vi "Event handler-Number of planes change.vi"(8 "error in (no error)":errorcluster) -> (0 "error out":errorcluster)   [LabVIEW 2020]
uses:
  Typedefs/Read Write Enum.ctl
  Global Variables/gl_UI Ctrl Refs.vi
  Global Variables/General Globals.vi
panel:
  out "Z-stop out (um)":dbl
  out "Z-start out (um)":dbl
  out "Adjusted absolute difference (um)":dbl
  out "Exact multiple?":bool
  out "Verified diffrence (um)":dbl
  out "Initial absolute difference (um)":dbl
  out "Z-stop (um)":dbl
  out "Z-start (um)":dbl
  out "Resulting Z Planes(um)":dbl[](array[numeric])
  out "Resulting number of planes":i32
  out "Z-step (um)":dbl
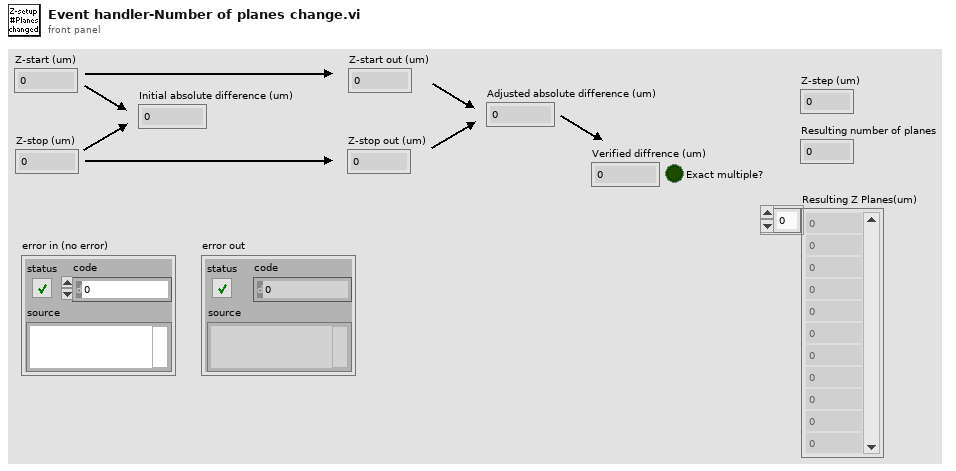
[diagram p1: front panel]
types:
  T1 = typedef "Read Write Enum.ctl" = enum16{"Read", "Write"}
  T2 = typedef "UI ctrl refs cluster.ctl" = cluster{"Top level VI path":path, "Top level VI ref":refnum<vi>, "User menu ref":refnum<k9>, "Sub Panel control":refnum<vi>, "Imaging Param Tab":refnum<vi>, "Occurrence-Start drivers":refnum<k4>, "Occurrence-Speed logging initialised":refnum<k4>, "Occurrence-XYZ stage initialised":refnum<k4>, "Exit button":refnum<vi>, "Status ind":refnum<vi>, "Set as origin":refnum<vi>, "Speed Logging":refnum<vi>, "Time Lapse":refnum<vi>, "Live Imaging":refnum<vi>, "AOL Z Stack":refnum<vi>, "Motor Z Stack":refnum<vi>, "Funct Acq button":refnum<vi>, "Hard Shutter":refnum<vi>, "Virtual Shutter":refnum<vi>, "Laser Power":refnum<vi>, "AOL Mode":refnum<vi>, "Frame Size":refnum<vi>, "Field of View":refnum<vi>, "Dwell Time":refnum<vi>, "Zoom":refnum<vi>, "AOL Z":refnum<vi>, "Objective":refnum<vi>, "Axis":refnum<vi>, "Paths & Names":refnum<vi>, "Experiment folder path (ind.)":refnum<vi>, "Last State (Ind.)":refnum<vi>, "Averages":refnum<vi>, "Angle (degrees)":refnum<vi>, "X centre":refnum<vi>, "Y centre":refnum<vi>, "Plane Mode":refnum<vi>, "# Planes":refnum<vi>, "Z Start":refnum<vi>, "Z Stop":refnum<vi>, "Z Step":refnum<vi>, "PMT 1":refnum<vi>, "PMT 2":refnum<vi>, "Stage XYZ Position":refnum<vi>, "Pockels@Z Start":refnum<vi>, "Pockels@Z Stop":refnum<vi>, "Obtain Z Start":refnum<vi>, "Obtain Z Stop":refnum<vi>, "Live stim.trig.period":refnum<vi>, "Live stim.trig.enable":refnum<vi>, "Movement Correction":refnum<vi>, "Load Reference Image":refnum<vi>, "XY Stage Move":refnum<vi>, "MovCor Cluster":refnum<vi>, "RefDAQParam":refnum<vi>, "Funct. Acq. Pockels Modulation":refnum<vi>, "Ref Laser Power":refnum<vi>, "Enable Video Recording":refnum<vi>, "Video Record-Live Imaging":refnum<vi>, "Video Record-Funct acq":refnum<vi>, "Reference Source":refnum<vi>, "AOL Z-stack Chirps Ready (ind)":refnum<vi>, "Target time between mov.cor. ref triggers (ms)":refnum<vi>, "Funct. Acq. Ref frame save":refnum<vi>, "Tracking button":refnum<vi>, "Show ref plots window":refnum<vi>, "Center freq ind (nm)":refnum<vi>, "Pickup mode (ind)":refnum<vi>, "Logging queue (ind)":refnum<vi>, "Back aperture power (ind.)":refnum<vi>, "Power after objective (ind.)":refnum<vi>, "Switch user":refnum<vi>, "Ls1 Conn. Status":refnum<vi>, "Ls1Tuning Status":refnum<vi>, "Ls1 Faults":refnum<vi>, "Ls1 Connection":refnum<vi>, "Ls1 Mode":refnum<vi>, "Ls1 POWER [mW]":refnum<vi>, "Ls1Shutter":refnum<vi>, "Ls1 Wavelength":refnum<vi>, "Ls1 Note":refnum<vi>, "Ls1 Confirm Wav":refnum<vi>, "Ls1 PreChrp Prism1":refnum<vi>, "Ls1 PreChrp Prism2":refnum<vi>, "Ls1 wav top Ind":refnum<vi>, "Ls1 power top Ind":refnum<vi>, "Ls1 Pump peak Hold":refnum<vi>, "Ls1 Status Ind":refnum<vi>, "Ls1 wav cancel":refnum<vi>, "Experiment Type":refnum<vi>, "Biology Information":refnum<vi>, "Camera recording status":refnum<vi>}
  T3 = cluster{"ZStack":cluster{"Zstart":dbl, "Zstop":dbl, "Zstep":dbl}, "Laser Power %":cluster{"@ Start":dbl, "@ Stop":dbl}}
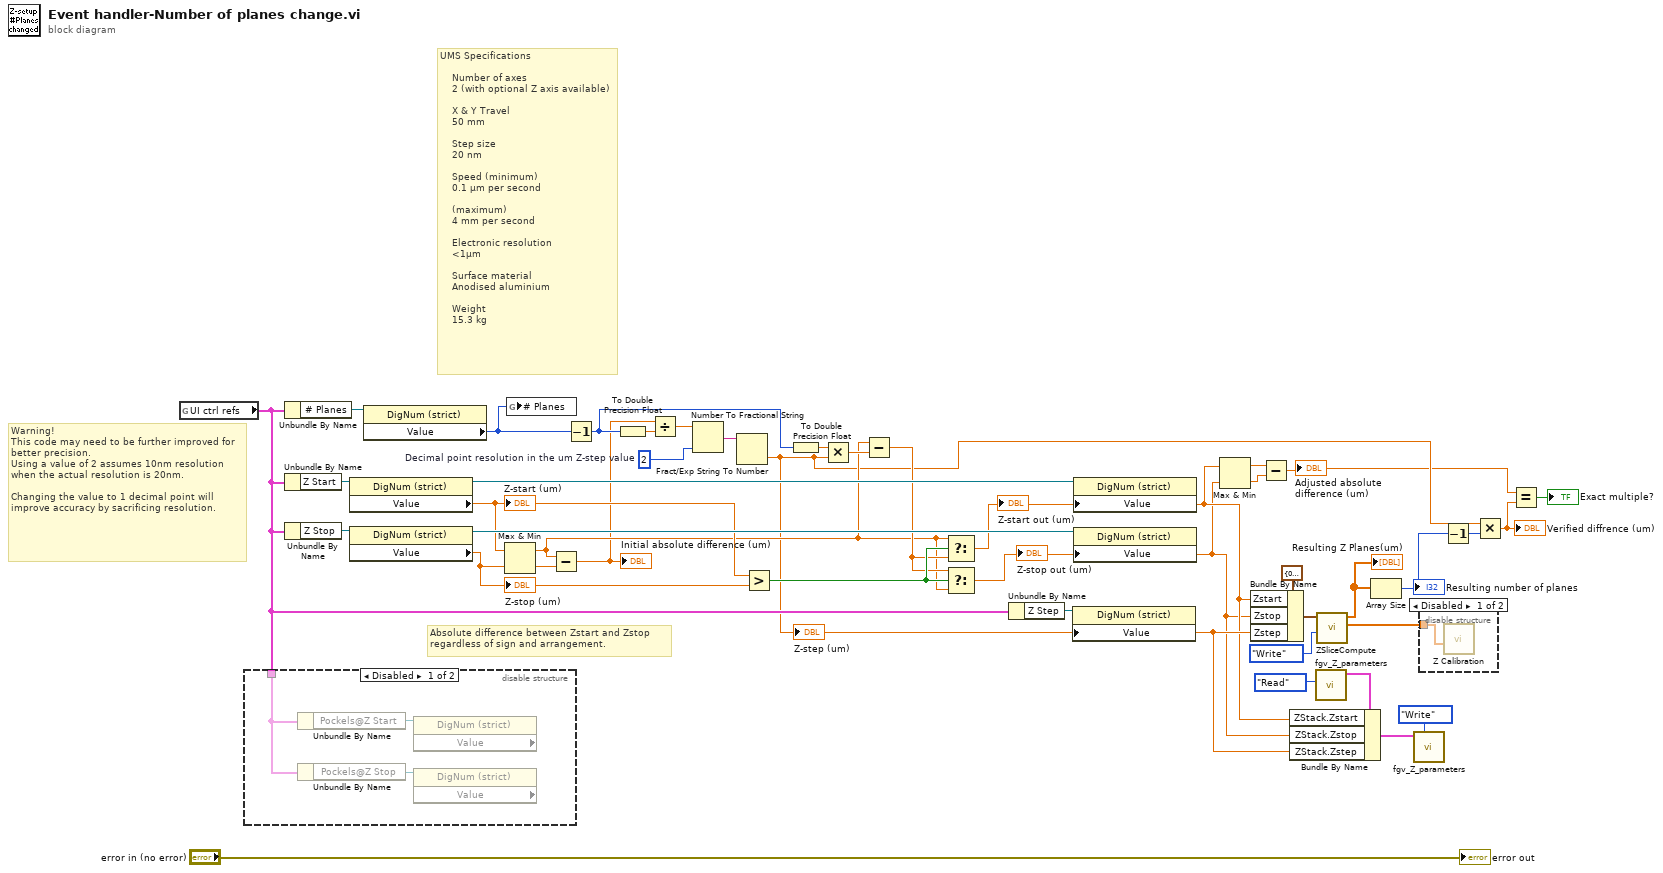
[diagram p0: block diagram]
diagram:
  w27 = i16 2  # Decimal point resolution in the um Z-step value
  # "Warning!\nThis code may need to be further improved for better precision.\nUsing a value of 2 assumes 10nm resolution when the actual resolution is 20nm.\n\nChanging the value to 1 decimal point will improve accuracy by sacrificing resolution."
  # "UMS Specifications\n\n    Number of axes\n    2 (with optional Z axis available)\n\n    X & Y Travel\n    50 mm\n\n    Step size\n    20 nm\n\n    Speed (minimum)\n    0.1 µm per second\n\n    (maximum)\n    4 mm per second\n\n    Electronic resolution\n    <1µm\n\n    Surface material\n    Anodised aluminium\n\n    Weight\n    15.3 kg"
  # "Absolute difference between Zstart and Zstop\nregardless of sign and arrangement."
  n1 = global read "gl_UI Ctrl Refs.vi" "UI ctrl refs"() -> (w42:T2)
  n2 = disable-structure shown="Disabled" {
    disable-tunnel: w42 -> [w45 _]
    frame Disabled {
      n3 = Unbundle By Name(w45) -> ("Pockels@Z Start"=w44:refnum<vi>)
      n4 = Unbundle By Name(w45) -> ("Pockels@Z Stop"=w43:refnum<vi>)
      n5 = property on="Property Node" class="DigNum (strict)" props=["Value"](reference=w44) -> ()  [unwired: 1 in, 3 out]
      n6 = property on="Property Node" class="DigNum (strict)" props=["Value"](reference=w43) -> ()  [unwired: 1 in, 3 out]
    }
    frame Enabled {
    }
  }
  n7 = Unbundle By Name(w42) -> ("# Planes"=w30:refnum<vi>)
  n8 = Unbundle By Name(w42) -> ("Z Start"=w33:refnum<vi>)
  n9 = Unbundle By Name(w42) -> ("Z Stop"=w32:refnum<vi>)
  n10 = property on="Property Node" class="DigNum (strict)"(reference=w33) -> (reference out=w17:refnum<vi>, "Value"=w18:dbl)  [unwired: 1 in, 1 out]
  "Z-start (um)" <- w18
  n11 = property on="Property Node" class="DigNum (strict)"(reference=w32) -> (reference out=w23:refnum<vi>, "Value"=w21:dbl)  [unwired: 1 in, 1 out]
  "Z-stop (um)" <- w21
  n12 = property on="Property Node" class="DigNum (strict)"(reference=w30) -> ("Value"=w2:u16)  [unwired: 1 in, 2 out]
  n13 = Max & Min(x=w18, y=w21) -> (max(x,y)=w14:dbl, min(x,y)=w19:dbl)
  n14 = global write "General Globals.vi" "# Planes"(w2) -> ()
  n15 = Subtract(x=w14, y=w19) -> (x-y=w8:dbl)
  "Initial absolute difference (um)" <- w8
  n16 = Decrement(x=w2) -> (x-1=w22:u16)
  n17 = To Double Precision Float(number=w22) -> (double precision float=w28:dbl)
  n18 = Divide(x=w8, y=w28) -> (x/y=w26:dbl)
  n19 = Number To Fractional String(number=w26, precision (6)=w27) -> (F-format string=w25:string)  [unwired: 2 in]
  n20 = Fract/Exp String To Number(string=w25) -> (number=w12:dbl)  [unwired: 3 in, 1 out]
  "Z-step (um)" <- w12
  n21 = Greater?(x=w18, y=w21) -> (0:w16:bool)
  n22 = To Double Precision Float(number=w22) -> (double precision float=w24:dbl)
  n23 = Multiply(x=w24, y=w12) -> (x*y=w20:dbl)
  n24 = Subtract(x=w14, y=w20) -> (x-y=w15:dbl)
  n25 = Select(t=w14, s=w16, f=w15) -> (s? t:f=w4:dbl)
  "Z-start out (um)" <- w4
  n26 = Select(t=w15, s=w16, f=w14) -> (s? t:f=w3:dbl)
  "Z-stop out (um)" <- w3
  n27 = Unbundle By Name(w42) -> ("Z Step"=w31:refnum<vi>)
  n28 = property on="Property Node" class="DigNum (strict)"(reference=w31, "Value"=w12) -> ()  [unwired: 1 in, 2 out]
  n29 = property on="Property Node" class="DigNum (strict)"(reference=w17, "Value"=w4) -> ()  [unwired: 1 in, 2 out]
  n30 = property on="Property Node" class="DigNum (strict)"(reference=w23, "Value"=w3) -> ()  [unwired: 1 in, 2 out]
  n31 = Max & Min(x=w4, y=w3) -> (max(x,y)=w7:dbl, min(x,y)=w6:dbl)
  n32 = Bundle By Name(cluster=cluster{"Zstart":dbl, "Zstop":dbl, "Zstep":dbl} {"Zstart"=0.0, "Zstop"=0.0, "Zstep"=0.0} ("ZStack"), "Zstart"=w4, "Zstop"=w3, "Zstep"=w12) -> (w40:cluster{"Zstart":dbl, "Zstop":dbl, "Zstep":dbl})
  n33 = Subtract(x=w7, y=w6) -> (x-y=w5:dbl)
  "Adjusted absolute difference (um)" <- w5
  n34 = call "fgv_Z_parameters.vi"("Function"=enum16{"Intialize", "Write", "Read", "Clear"}."Read") -> ("Z Parameters"=w35:T3)  [unwired: 9 in, 1 out]
  n35 = Bundle By Name(cluster=w35, "ZStack.Zstart"=w4, "ZStack.Zstop"=w3, "ZStack.Zstep"=w12) -> (w34:T3)
  n36 = call "ZSliceCompute.vi"("Function"=Read_Write_Enum."Write", "ZStack (um)"=w40) -> ("AOL Z Planes(um)"=w38:dbl[], "Motor Z Planes(um)"=w39:dbl[])  [unwired: 6 in, 2 out]
  "Resulting Z Planes(um)" <- w39
  n37 = Array Size(array=w39) -> (size(s)=w13:i32)
  "Resulting number of planes" <- w13
  n38 = call "fgv_Z_parameters.vi"("Function"=enum16{"Intialize", "Write", "Read", "Clear"}."Write", "Z Parameters"=w34) -> ()  [unwired: 8 in, 2 out]
  n39 = disable-structure "Diagram Disable Structure" shown="Disabled" {
    disable-tunnel: w38 -> [w46 _]
    frame Disabled {
      n40 = call "Z Calibration.vi"("Z Planes"=w46) -> ()  [unwired: 7 in, 4 out]
    }
    frame Enabled {
    }
  }
  n41 = Decrement(x=w13) -> (x-1=w11:i32)
  n42 = Multiply(x=w12, y=w11) -> (x*y=w10:dbl)
  "Verified diffrence (um)" <- w10
  n43 = Equal?(x=w5, y=w10) -> (x = y?=→"Exact multiple?":bool)
  "error out" <- "error in (no error)"
